vi "Setup UI.vi"(8 "error in (no error)":errorcluster, 11 "Operator UI in":refnum<class "Controller UI.lvclass">) -> (0 "error out":errorcluster, 3 "Operator UI out":refnum<class "Controller UI.lvclass">)   [LabVIEW 2016, in "Controller UI.lvlib" / "Controller UI.lvclass"]
uses:
  <userlib>/Common Components/Controller UI/Controller UI.lvclass
  <userlib>/Common Components/Controller UI/Controller UI.lvclass/Controller UI.ctl
  <vilib>/Utility/miscctls.llb/LVRowAndColumnTypeDef.ctl
  <vilib>/Utility/miscctls.llb/LVRowAndColumnUnsignedTypeDef.ctl
  <userlib>/Common Components/Controller UI/Accessors/Read Show FP_.vi
  <userlib>/Common Components/Controller UI/Accessors/Read Status Display.vi
  <userlib>/Common Components/Controller UI/Accessors/Read Results Listbox.vi
  <userlib>/Common Components/Controller UI/Accessors/Read View Results.vi
  <userlib>/Common Components/Controller UI/Accessors/Read Tab Control.vi
  <userlib>/Common Components/Controller UI/Accessors/Read Run.vi
  <userlib>/Common Components/Controller UI/Accessors/Read Function.vi
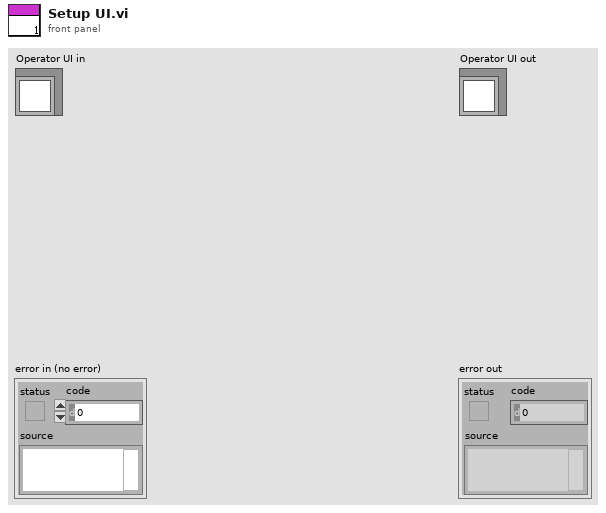
[diagram p1: front panel]
types:
  T1 = enum8{"Enabled", "Disabled", "Disabled and Grayed Out"}
  T2 = typedef "LVRowAndColumnUnsignedTypeDef.ctl" = cluster{"Row":u32, "Column":u32}
  T3 = typedef "LVRowAndColumnTypeDef.ctl" = cluster{"Row":i32, "Column":i32}
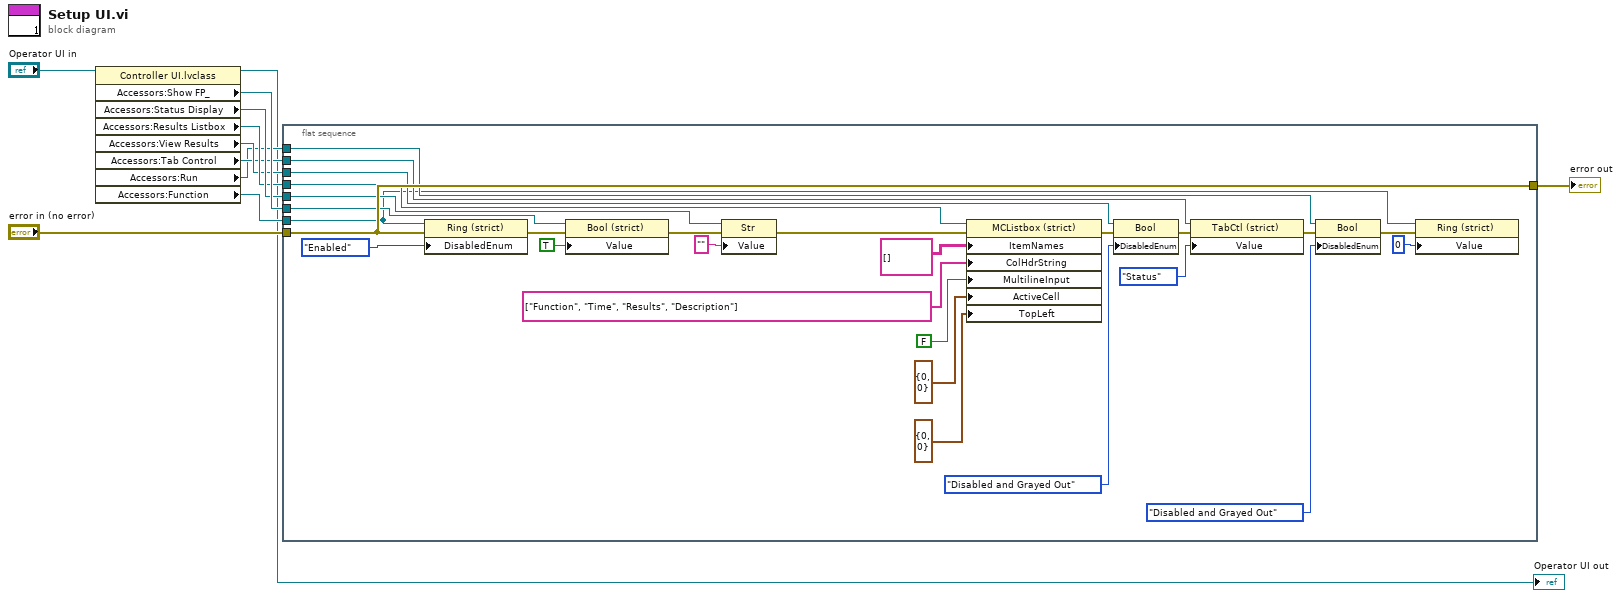
[diagram p0: block diagram]
diagram:
  n1 = property class="Controller UI.lvclass"(reference="Operator UI in") -> (reference out=→"Operator UI out":refnum<class "Controller UI.lvclass">, "Accessors:Show FP_"=w9:refnum<vi>, "Accessors:Status Display"=w8:refnum<vi>, "Accessors:Results Listbox"=w7:refnum<vi>, "Accessors:View Results"=w6:refnum<vi>, "Accessors:Tab Control"=w5:refnum<vi>, "Accessors:Run"=w4:refnum<vi>, "Accessors:Function"=w3:refnum<vi>)  [unwired: 1 in, 1 out]
  n2 = flat-sequence {
    tunnel: "error in (no error)" -> [w23]
    tunnel: [w23] -> w2
    tunnel: w9 -> [w21]
    tunnel: w8 -> [w20]
    tunnel: w7 -> [w19]
    tunnel: w6 -> [w18]
    tunnel: w5 -> [w17]
    tunnel: w4 -> [w16]
    tunnel: w3 -> [w15]
    frame #0 {
      n3 = property class="Ring (strict)"(reference=w15, error in=w23, "DisabledEnum"=T1."Enabled" ("Disabled")) -> (error out=w22:errorcluster)  [unwired: 1 out]
      n4 = property class="Bool (strict)"(reference=w21, error in=w22, "Value"=TRUE) -> (error out=w29:errorcluster)  [unwired: 1 out]
      n5 = property class="Str"(reference=w20, error in=w29, "Value"="") -> (error out=w14:errorcluster)  [unwired: 1 out]
      n6 = property class="MCListbox (strict)"(reference=w19, error in=w14, "ItemNames"=string[][] [] ("Item Names"), "ColHdrString"=string[] ["Function", "Time", "Results", "Description"] ("Column Header Strings[]"), "MultilineInput"=FALSE ("Multiple Line Input"), "ActiveCell"=T3 {"Row"=0, "Column"=0} ("Active Cell:Active Cell"), "TopLeft"=T2 {"Row"=0, "Column"=0} ("Top Left Visible Cell")) -> (error out=w30:errorcluster)  [unwired: 1 out]
      n7 = property class="Bool"(reference=w18, error in=w30, "DisabledEnum"=T1."Disabled and Grayed Out" ("Disabled")) -> (error out=w13:errorcluster)  [unwired: 1 out]
      n8 = property class="TabCtl (strict)"(reference=w17, error in=w13, "Value"=enum32{"Status", "Results"}."Status") -> (error out=w12:errorcluster)  [unwired: 1 out]
      n9 = property class="Bool"(reference=w16, error in=w12, "DisabledEnum"=T1."Disabled and Grayed Out" ("Disabled")) -> (error out=w31:errorcluster)  [unwired: 1 out]
      n10 = property class="Ring (strict)"(reference=w15, error in=w31, "Value"=u16 0) -> ()  [unwired: 2 out]
    }
  }
  "error out" <- w2
